vi "analog gas detector using thingpings.vi"() -> ()   [LabVIEW 2021]
uses:
  <vilib>/MakerHub/LINX/Public/Peripherals/Analog/Analog Read 1 Chan.vi
  <vilib>/MakerHub/LINX/Public/Peripherals/Analog/Analog Read N Chans.vi
  <vilib>/MakerHub/LINX/Private/Local IO/LinxAnalogRead.vi
  <vilib>/MakerHub/LINX/Public/Utilities/Check Channel.vi
  <vilib>/MakerHub/LINX/Public/Utilities/Open Serial.vi
  <vilib>/MakerHub/LINX/Private/Utilties/Generate Error.vi
  <vilib>/MakerHub/LINX/LMH-LINX.lvlib
  <vilib>/httpClient/LabVIEWHTTPClient.lvlib
panel:
  in  "stop":bool
  out "Voltage":dbl
  in  "Serial Port":refnum<visa-resource-name>="N/A"
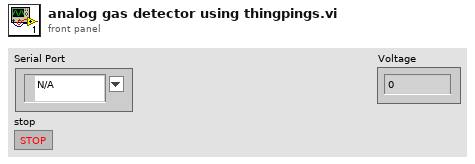
[diagram p1: front panel]
types:
  T1 = typedef "LMH-LINX.lvlib/LINX Ref.ctl" = cluster{"IO":T2, "Interface":T3, "LINX Device Config":T4}
  T2 = typedef "LMH-LINX.lvlib/Platform.ctl" = enum16{"Remote", "Local"}
  T3 = typedef "LMH-LINX.lvlib/Interface.ctl" = enum16{"Serial", "TCP"}
  T4 = typedef "LMH-LINX.lvlib/Device.lvlib/LINX Device Config.ctl" = cluster{"Interface":T3, "COM Port":refnum<visa-resource-name>, "TCP Configuration":T5, "Device Family":u8, "Device ID":u8, "Device Name":string, "TCP Ref":refnum<k5>, "Channels":T6}
  T5 = typedef "LMH-LINX.lvlib/Device.lvlib/TCP Config.ctl" = cluster{"IP Address":string, "Port":u16}
  T6 = typedef "LMH-LINX.lvlib/Channels.ctl" = cluster{"DI":u8[], "DO":u8[], "AI":u8[], "AO":u8[], "PWM":u8[], "QE":u8[], "UART":u8[], "I2C 2":u8[], "SPI":u8[], "CAN":u8[], "Servo":u8[], "AI Ref (V)":dbl, "AI Resolution (Bits)":u8, "AO Ref (V)":dbl, "AO Resolution (Bits)":u8}
  T7 = typedef "LabVIEWHTTPClient.lvlib/ClientHandle.ctl" = refnum<k1>
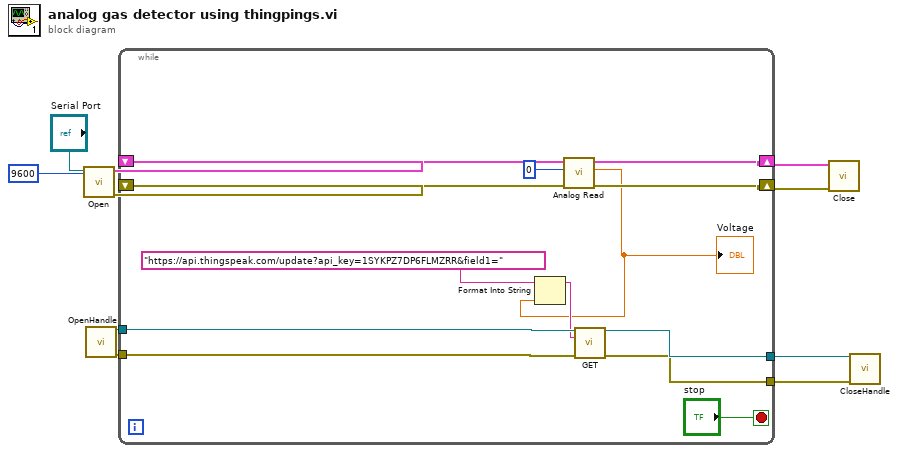
[diagram p0: block diagram]
diagram:
  n1 = call-poly <vilib>:"Open.vi"("Baud Rate Override"=u32 9600, "Serial Port"="Serial Port") -> ("Error Out"=w8:errorcluster, "LINX Resource"=w10:T1)  [unwired: 7 in, 1 out]
  n2 = call <vilib>:"OpenHandle.vi"() -> ("client handle out"=w4:T7, "error out"=w2:errorcluster)  [unwired: 14 in]
  n3 = while {
    shift-right: [w22] -> w9
    shift-left: w10 -> [w23]
    shift-right: [w20] -> w7
    shift-left: w8 -> [w21]
    tunnel: w4 -> [w17]
    tunnel: [w16] -> w3
    tunnel: w2 -> [w15]
    tunnel: [w14] -> w1
    stop <- "stop" stop-if-true
    n4 = call-poly <vilib>:"Analog Read.vi"("Error In"=w21, "Analog Channel"=u8 0, "LINX Resource"=w23) -> ("Error Out"=w20:errorcluster, "Voltage"=w11:dbl, "LINX Resource"=w22:T1)  [unwired: 5 in, 1 out]
    "Voltage" <- w11
    n5 = Format Into String(initial string="https://api.thingspeak.com/update?api_key=1SYKPZ7DP6FLMZRR&field1=" ("url"), w11) -> (resulting string=w12:string)  [unwired: 2 in, 1 out]
    n6 = call <vilib>:"GET.vi"("client handle"=w17, "url"=w12, "error in (no error)"=w15) -> ("client handle out"=w16:T7, "error out"=w14:errorcluster)  [unwired: 9 in, 2 out]
  }
  n7 = call <vilib>:"Close.vi"("Error In"=w7, "LINX Resource"=w9) -> ()  [unwired: 9 in, 1 out]
  n8 = call <vilib>:"CloseHandle.vi"("client handle"=w3, "error in (no error)"=w1) -> ()  [unwired: 13 in, 1 out]
